vi "dspic.vi"() -> ()   [LabVIEW 2020]
uses:
  <vilib>/Instr/_visa.llb/VISA Configure Serial Port (Instr).vi
panel:
  out "error out":errorcluster
  out "serial":refnum<visa-resource-name>
  in  "Tab Control":enum32{"DASHBOARD"}(tab)
  out "W":dbl(knob) scale=0.0..210.0
  in  "GIRO":bool
  out "DATA":T1(graph)
  in  "SET POINT":dbl(knob) scale=0.0..220.0
  out "VELOCIDAD ANGULAR":string
  in  "Puerto Serial":refnum<visa-resource-name>
  in  "STOP":bool
  # "CONTROL PID - dsPIC"
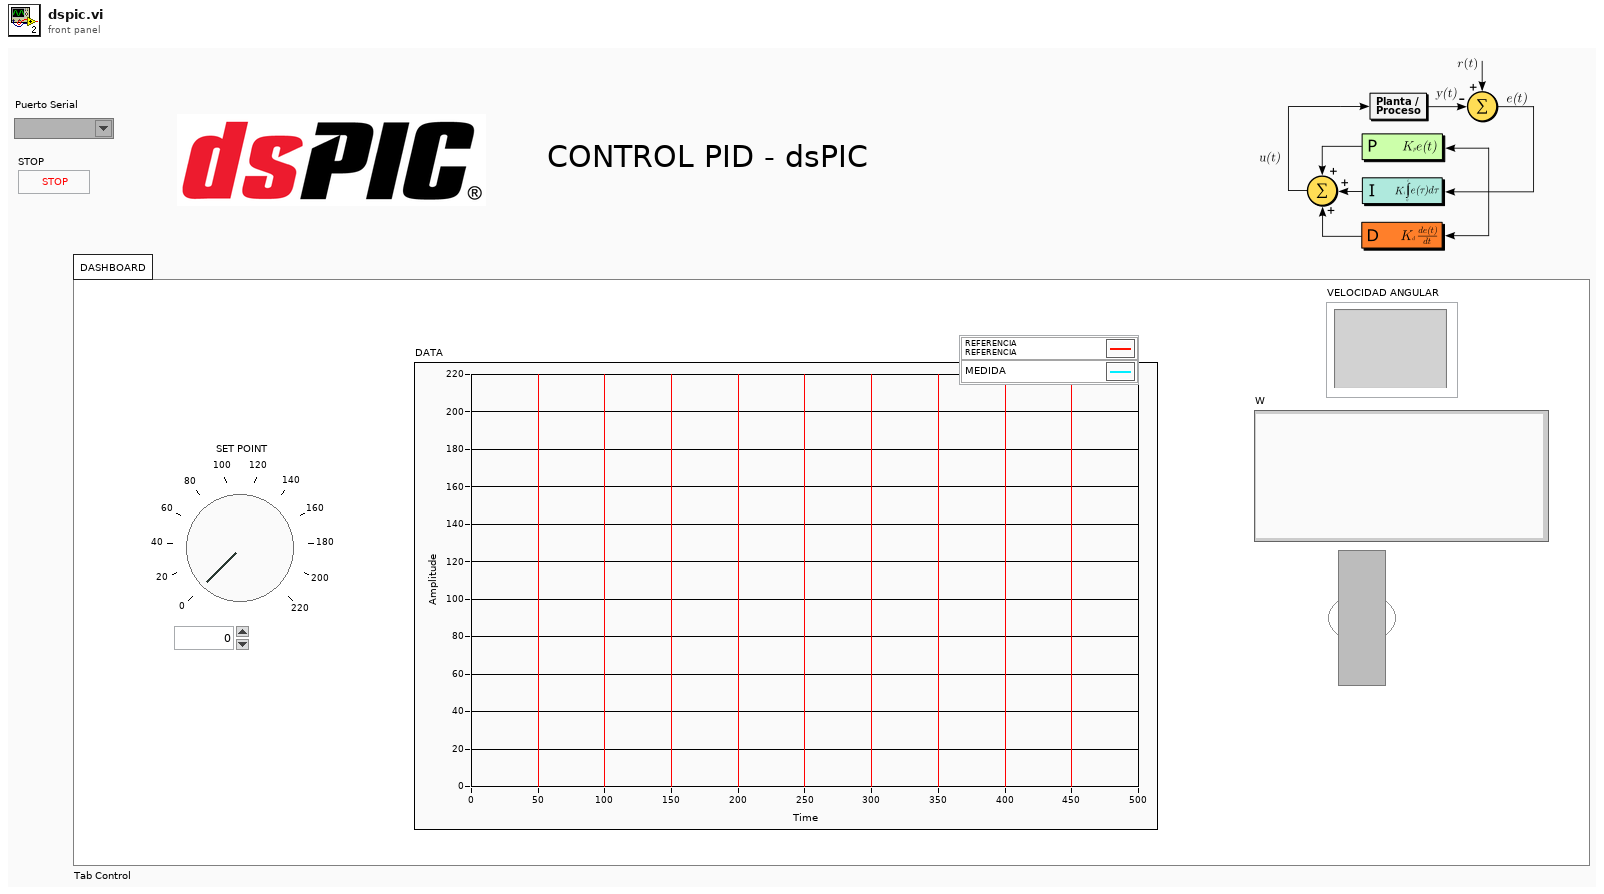
[diagram p1: front panel]
types:
  T1 = cluster{"[0]":dbl, "[1]":dbl, "[2]":dbl, "[3]":dbl, "[4]":dbl, "[5]":dbl, "[6]":dbl, "[7]":dbl, "[8]":dbl}
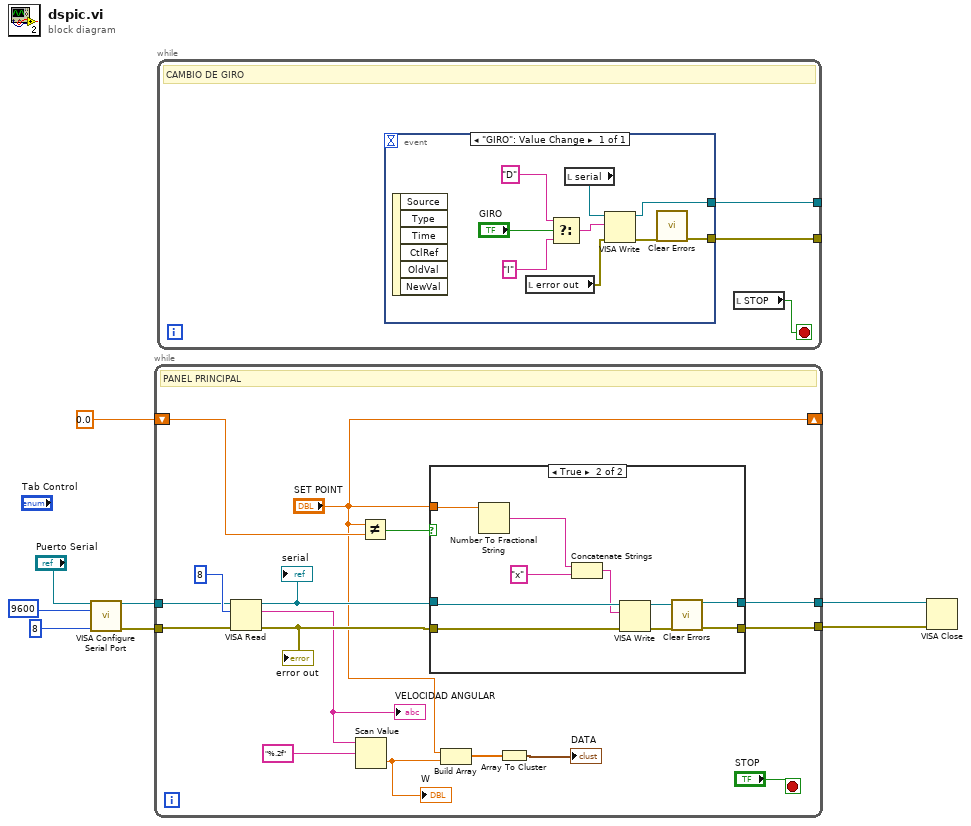
[diagram p0: block diagram]
diagram:
  n1 = call-poly "VISA Configure Serial Port"("VISA resource name"="Puerto Serial", "baud rate (9600)"=u32 9600, "data bits (8)"=u16 8) -> ("VISA resource name out"=w5:refnum<visa-resource-name>, "error out"=w6:errorcluster)  [unwired: 11 in]
  n2 = while {
    tunnel: w6 -> [w11]
    tunnel: w5 -> [w12]
    tunnel: [w23] -> w4
    tunnel: [w22] -> w3
    shift-right: ["SET POINT"] -> _
    shift-left: 0.0 -> [w20]
    stop <- "STOP" stop-if-true
    # "PANEL PRINCIPAL"
    n3 = VISA Read(VISA resource name=w12, byte count=u32 8, error in (no error)=w11) -> (VISA resource name out=w15:refnum<visa-resource-name>, read buffer=w10:string, error out=w14:errorcluster)  [unwired: 1 out]
    "VELOCIDAD ANGULAR" <- w10
    "serial" <- w15
    "error out" <- w14
    n4 = Scan Value(string=w10, format string="%.2f") -> (value=w13:dbl)  [unwired: 1 in, 1 out]
    "W" <- w13
    n5 = Not Equal?(x="SET POINT", y=w20) -> (x != y?=w21:bool)
    n6 = case shown="True" w21 {
      tunnel: "SET POINT" -> [_ w35]
      tunnel: w15 -> [w26 w34]
      tunnel: w14 -> [w25 w33]
      tunnel: [w25 w31] -> w23
      tunnel: [w26 w30] -> w22
      frame False {
      }
      frame True {
        n7 = Number To Fractional String(number=w35) -> (F-format string=w29:string)  [unwired: 3 in]
        n8 = Concatenate Strings(w29, "x" ("string")) -> (w28:string)
        n9 = VISA Write(VISA resource name=w34, write buffer=w28, error in (no error)=w33) -> (VISA resource name out=w30:refnum<visa-resource-name>, error out=w32:errorcluster)  [unwired: 1 out]
        n10 = call <vilib>:"Clear Errors.vi"("error in (no error)"=w32) -> ("error out"=w31:errorcluster)  [unwired: 5 in, 1 out]
      }
    }
    n11 = Build Array("SET POINT", w13) -> (w18:dbl[])
    n12 = Array To Cluster(array=w18) -> (cluster=→"DATA":T1)
  }
  n13 = while {
    tunnel: [w38] -> _
    tunnel: [w37] -> _
    stop <- w36 stop-if-true
    # "CAMBIO DE GIRO"
    n14 = event shown="[0] \"GIRO\": Value Change" {
      selector: _ -> [_]
      dyn-events: _ -> [_]
      timeout: _ -> [_]
      tunnel: [w43] -> w38
      tunnel: [w42] -> w37
      event "GIRO": Value Change {
        n15 = event-data() -> ()  [unwired: 1 in, 6 out]
        n16 = local read "error out"() -> (w39:errorcluster)
        n17 = Select(t="D", s="GIRO", f="I") -> (s? t:f=w41:string)
        n18 = local read "serial"() -> (w40:refnum<visa-resource-name>)
        n19 = VISA Write(VISA resource name=w40, write buffer=w41, error in (no error)=w39) -> (VISA resource name out=w43:refnum<visa-resource-name>, error out=w44:errorcluster)  [unwired: 1 out]
        n20 = call <vilib>:"Clear Errors.vi"("error in (no error)"=w44) -> ("error out"=w42:errorcluster)  [unwired: 5 in, 1 out]
      }
    }
    n21 = local read "STOP"() -> (w36:bool)
  }
  n22 = VISA Close(VISA resource name=w3, error in (no error)=w4) -> ()  [unwired: 1 out]
